vi "Get Horizontal Offset Limits.vi"(0 "rx output divider":T1, 11 "error in":errorcluster) -> (4 "maximum":i16, 6 "minimum":i16, 8 "number of horizontal points":i16, 15 "error out":errorcluster)   [LabVIEW 2015, in "niHighSpeedSerial Eye Scan Common v1 Host.lvlib"]
uses:
  <instrlib>/niHighSpeedSerial/Eye Scan/v1/Host/Common/niHighSpeedSerial Eye Scan Common v1 Host.lvlib
  <instrlib>/niHighSpeedSerial/Eye Scan/v1/Host/Common/Public/RX Output Divider.ctl
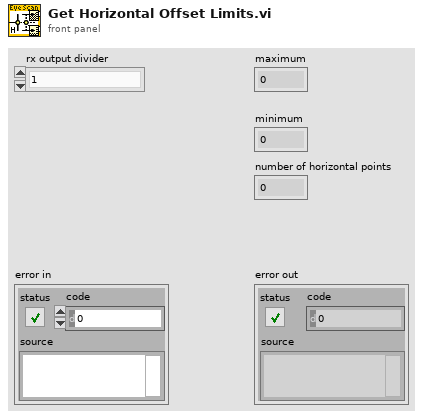
[diagram p1: front panel]
types:
  T1 = typedef "niHighSpeedSerial Eye Scan Common v1 Host.lvlib/RX Output Divider.ctl" = enum16{"1", "2", "4", "8", "16"}
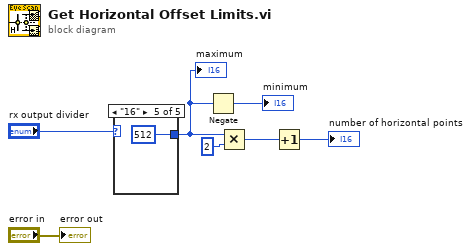
[diagram p0: block diagram]
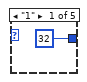
[diagram p2: hidden frame]
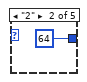
[diagram p3: hidden frame]
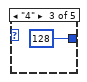
[diagram p4: hidden frame]
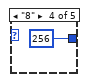
[diagram p5: hidden frame]
diagram:
  n1 = case shown="\"16\"" "rx output divider" {
    tunnel: [i16 32 ("upper limit") i16 64 ("upper limit") i16 128 ("upper limit") i16 256 ("upper limit") i16 512 ("upper limit")] -> w4
    frame "1" {
    }
    frame "2" {
    }
    frame "4" {
    }
    frame "8" {
    }
    frame "16" {
    }
  }
  "maximum" <- w4
  n2 = Negate(x=w4) -> (-x=→"minimum":i16)
  n3 = Multiply(x=w4, y=i16 2) -> (x*y=w2:i16)
  n4 = Increment(x=w2) -> (x+1=→"number of horizontal points":i16)
  "error out" <- "error in"
